vi "TEST - Size of Data from TD.vi"(8 "error in (no error)":errorcluster) -> (0 "error out":errorcluster, 2 "Pass":bool)   [LabVIEW 2020, in "test_openg_variant.lvlib"]
uses:
  test_openg_variant.lvlib
  <userlib>/_OpenG.lib/error/error.llb/openg_error.lvlib
  source/library/openg_variant.lvlib
  source/library/Type Descriptor.ctl
panel:
  out "Failures":T2(array[cluster])
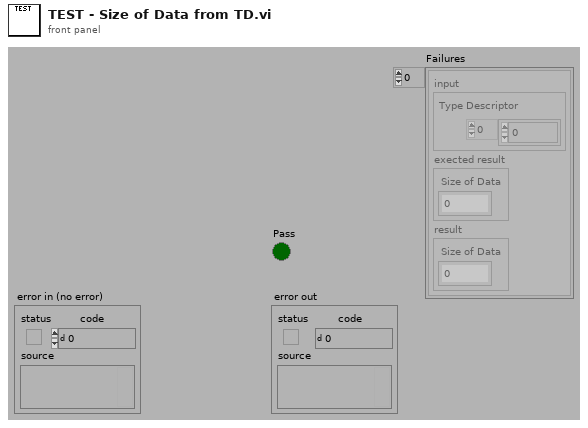
[diagram p1: front panel]
types:
  T1 = typedef "openg_variant.lvlib/Type Descriptor.ctl" = i16[]
  T2 = cluster{"input":cluster{"Type Descriptor":T1}, "exected result":cluster{"Size of Data":i32}, "result":cluster{"Size of Data":i32}}[]
  T3 = cluster{"input":cluster{"Type Descriptor":T1}, "exected result":cluster{"Size of Data":i32}, "result":cluster{"Size of Data":i32}}
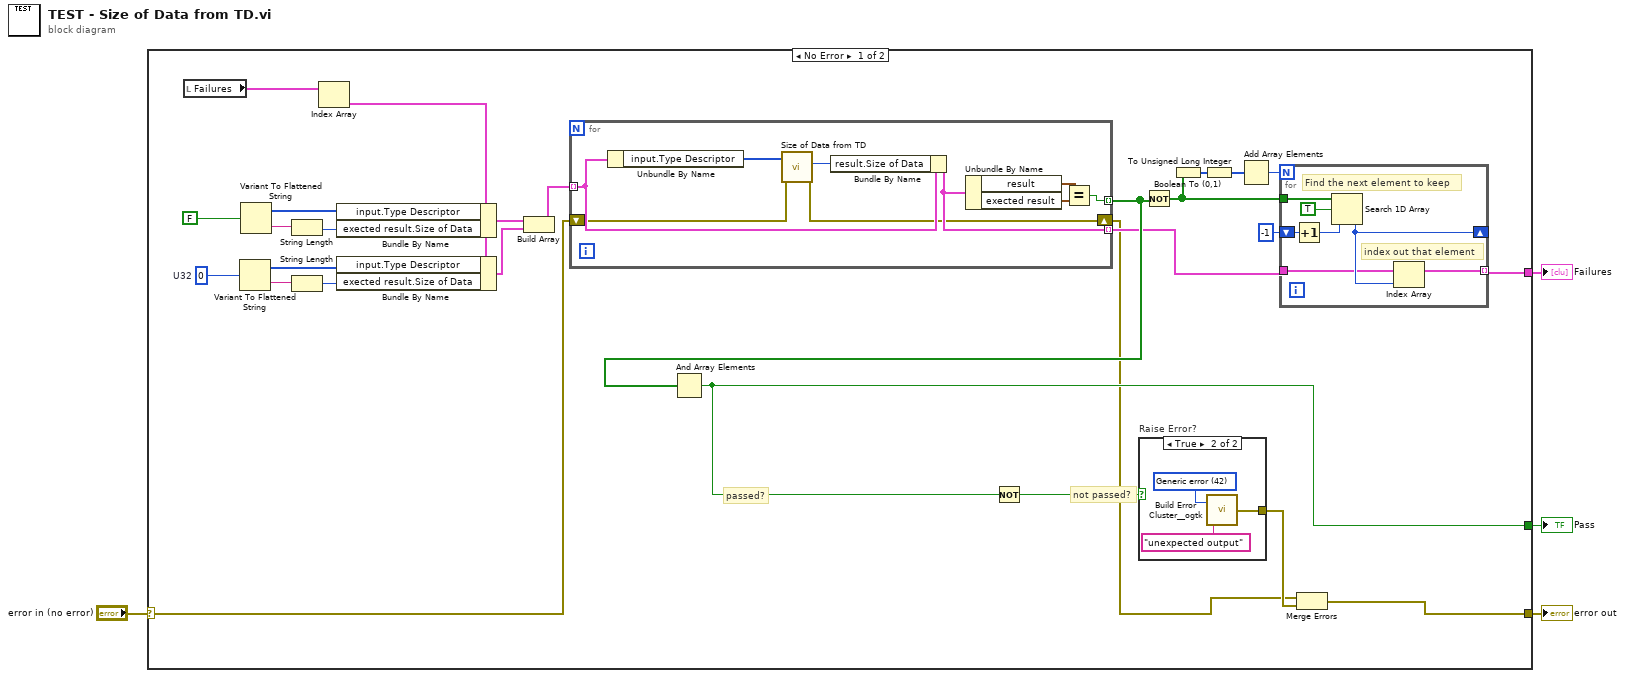
[diagram p0: block diagram]
diagram:
  n1 = case shown="No Error" "error in (no error)" {
    selector: "error in (no error)" -> [w17 w51]
    tunnel: [w28 _] -> w4
    tunnel: [w31 w51] -> w2
    tunnel: [w20 _] -> w1
    frame No Error {
      w5 = u32 0  # U32
      # "not passed?"
      # "passed?"
      n2 = local read "Failures"() -> (w15:T2)
      n3 = Variant To Flattened String(Variant=w5) -> (data string=w6:string, 1:w7:i16[])
      n4 = Variant To Flattened String(Variant=FALSE) -> (data string=w9:string, 1:w10:i16[])
      n5 = String Length(string=w9) -> (length=w14:i32)
      n6 = String Length(string=w6) -> (length=w13:i32)
      n7 = Index Array(array=w15) -> (element=w11:T3)  [unwired: 1 in]
      n8 = Bundle By Name(cluster=w11, "input.Type Descriptor"=w10, "exected result.Size of Data"=w14) -> (w19:T3)
      n9 = Bundle By Name(cluster=w11, "input.Type Descriptor"=w7, "exected result.Size of Data"=w13) -> (w12:T3)
      n10 = Build Array(w19, w12) -> (w18:T2)
      n11 = for {
        tunnel: w18 -> [w46] mode=indexing
        tunnel: [w47] -> w22 mode=indexing
        tunnel: [w45] -> w21 mode=indexing
        shift-right: [w41] -> w16
        shift-left: w17 -> [w42]
        n12 = Unbundle By Name(w46) -> ("input.Type Descriptor"=w40:T1)
        n13 = call "Size of Data from TD.vi"("error in (no error)"=w42, "Type Descriptor"=w40) -> ("error out"=w41:errorcluster, "Size of Data"=w39:i32)  [unwired: 8 in]
        n14 = Bundle By Name(cluster=w46, "result.Size of Data"=w39) -> (w45:T3)
        n15 = Unbundle By Name(w45) -> ("result"=w44:cluster{"Size of Data":i32}, "exected result"=w43:cluster{"Size of Data":i32})
        n16 = Equal?(x=w44, y=w43) -> (x = y?=w47:bool)
      }
      n17 = And Array Elements(Boolean array=w22) -> (logical AND=w28:bool)
      n18 = Not(x=w28) -> (.not. x?=w29:bool)
      n19 = case "Raise Error?" shown="True" w29 {
        tunnel: [_ w48] -> w30
        frame False {
        }
        frame True {
          w49 = 42 items=["No error", "Argument error", "Memory is full", "Out of zone", "End of file", "File already open", "Generic file I/O error", "File not found", "File permission error", "Disk is full", "Duplicate path", "Too many files open", "System feature not enabled", "Resource file not found", "Cannot add resource", "Resource not found", "Image not found", "Image memory error", "Pen does not exist", "Config type invalid", "Config token not found", "Config parse error", "Config memory error", "Bad external code format", "Bad external code offset", "External code not present", "Null window", "Destroy window error", "Null menu", "Print aborted", "Bad print record", "Print driver error", "Windows error during printing", "Memory error during printing", "Print dialog error", "Generic print error", "Invalid device refnum", "Device not found", "Device parameter error", "Device unit error", "Cannot open device", "Device call aborted", "Generic error", "Cancelled by user", "Object ID too low", "Object ID too high", "Object not in heap", "Unknown heap", "Unknown object (invalid DefProc)", "Unknown object (DefProc not in table)", "Message out of range", "Invalid (null) method", "Unknown message", "Manager call not supported", "Bad address", "Network operation in progress", "Network operation timed out", "Connection is busy", "Network attribute not supported", "Network error", "Address in use", "System out of memory", "Connection aborted", "Connection refused", "Not connected", "Already connected", "Connection closed", "Initialization error (interapplication manager)", "Bad occurrence", "Wait on unbound occurrence handler", "Occurrence queue overflow", "Datalog type conflict", "Unused", "Unrecognized type (interapplication manager)", "Memory corrupt", "Failed to make temporary DLL", "Old CIN version", "Drag socket not found", "Failed to load drop-object", "Failed to register OLE object", "Failed to release OLE object", "Format specifier type mismatch", "Unknown format specifier", "Too few format specifiers", "Too many format specifiers", "Scan failed", "Newer CIN version", "Error converting to variant", "Runtime menu error", "Password tampered", "Variant attribute not found", "Incompatible variant data type", "Event data is not available", "Event Store is not present", "Occurrence is not found", "Event Queue is not created", "Event info is not available", "Refnum passed is NULL", "Error retrieving Class GUID", "Error retrieving CoClass GUID", "Error retrieving TypeLib GUID.", "Bad built application magic bytes.", "Specific driver is different from the specific driver associated with the Logical Name.", "There is no session opened to the class driver.", "Max Error", "MAX - Error with config objects", "MAX - Error loading configuration", "MAX - Group not supported"]
          n20 = call <userlib>:"Build Error Cluster__ogtk.vi"("String to Prepend to source (\"\")"="unexpected output" ("String to Prepend to source (\"\")"), "code"=w49) -> ("error out"=w48:errorcluster)
        }
      }
      n21 = Not(x=w22) -> (.not. x?=w24:bool[])
      n22 = Boolean To (0,1)(Boolean=w24) -> (0, 1=w25:i16[])
      n23 = To Unsigned Long Integer(number=w25) -> (unsigned 32bit integer=w23:u32[])
      n24 = Add Array Elements(numeric array=w23) -> (sum=w26:u32)
      n25 = for {
        N: w26 -> [_]
        tunnel: w21 -> [w34]
        tunnel: w24 -> [w38]
        shift-right: [w35] -> _
        shift-left: -1 ("start index (0)") -> [w36]
        tunnel: [w33] -> w20 mode=indexing
        # "index out that element"
        # "Find the next element to keep"
        n26 = Increment(x=w36) -> (x+1=w32:i32)
        n27 = Search 1D Array(1D array=w38, element=TRUE, start index (0)=w32) -> (index of element=w35:i32)
        n28 = Index Array(array=w34, index=w35) -> (element=w33:T3)
      }
      n29 = Merge Errors(w16, w30) -> (w31:errorcluster)
    }
    frame Error {
    }
  }
  "Pass" <- w4
  "error out" <- w2
  "Failures" <- w1
